vi "ScanCtrl_TE.vi"() -> ()   [LabVIEW 2024]
uses:
  SubVI/GRBL/Status.ctl
  <vilib>/event_ctls.llb/usereventprio.ctl
  <vilib>/ErrorRing/Error Ring.xnode
  SubVI/GRBL/GRBL 1.1.lvlib
panel:
  out "error out":errorcluster
  in  "AutoStartFLIm?":bool
  out "Stage":bool
  in  "Save Button":bool
  in  "RasterScan":bool
  in  "Pre Scan Speed (mm/min)":sgl=3000.0
  in  "Y Pixel Size(mm)":dbl=1.0
  in  "Y distance(mm)":dbl=10.0
  in  "X distance (mm)":dbl=10.0
  in  "Stage COM port":refnum<visa-resource-name>="COM7"
  in  "Tab Control":enum32{"Stage Control", "Stage Setting"}(tab)
  out "Scan Origin MPos":cluster{"X":sgl, "Y":sgl, "Z":sgl}
  in  "Set Origin":bool
  in  "Jog Step Size(mm)":dbl=5.0
  in  "Z--":bool
  in  "Z++":bool
  in  "Y--":bool
  in  "Y++":bool
  in  "X--":bool
  in  "X++":bool
  in  "Hault":bool
  in  "Home":bool
  in  "GoToZero":bool
  out "Current Machine Pos":cluster{"X":sgl, "Y":sgl, "Z":sgl}
  in  "Poll grbl position?":bool
  out "Stage Home MPos":cluster{"X":sgl, "Y":sgl, "Z":sgl}
  in  "X-Axis configuration":T1={"Travel resolution\t(step/mm)"=160.0, "Maximum rate\t(mm/min)"=6000, "Acceleration\t(mm/sec^2)"=1000, "Maximum travel\t(mm)"=160}
  in  "Y-Axis configuration":T1={"Travel resolution\t(step/mm)"=160.0, "Maximum rate\t(mm/min)"=2000, "Acceleration\t(mm/sec^2)"=250, "Maximum travel\t(mm)"=160}
  in  "Z-Axis configuration":T1={"Travel resolution\t(step/mm)"=160.0, "Maximum rate\t(mm/min)"=2000, "Acceleration\t(mm/sec^2)"=250, "Maximum travel\t(mm)"=160}
  out "Current Config":string="$0=10\r\n$1=255\r\n$2=0\r\n$3=0\r\n$4=0\r\n$5=1\r\n$6=0\r\n$10=1\r\n$11=0.010\r\n$12=1000.000\r\n$13=0\r\n$20=1\r\n$21=0\r\n$22=1\r\n$23=0\r\n$24=5.000\r\n$25=3000.000\r\n$26=25\r\n$27=2.000\r\n$30=12000\r\n$31=4000\r\n$32=0\r\n$100=13.333\r\n$101=13.333\r\n$102=98.000\r\n$110=50000.000\r\n$111=50000.000\r\n$112=1800.000\r\n$120=250.000\r\n$121=250.000\r\n$122=50.000\r\n$130=267.000\r\n$131=472.000\r\n$132=68.000\r\nok\r\nok\r\n"
  out "Version information":string="[VER:1.1f.20170324:]\r\n[OPT:VM,15,128]\r\nok\r\nok\r\n"
  in  "Quit":bool
  # "3D Profile Scan Setting"
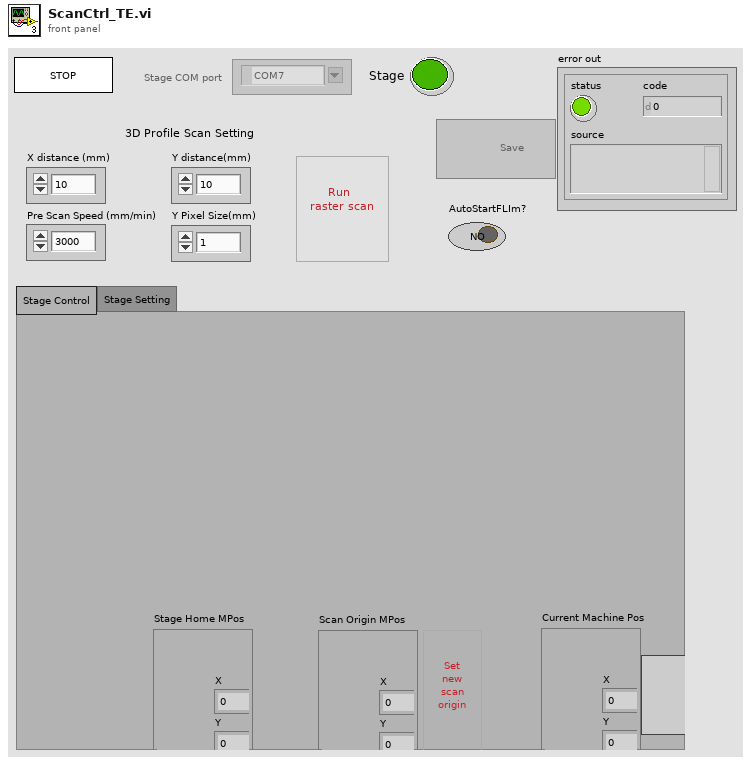
[diagram p1: front panel]
types:
  T1 = cluster{"Travel resolution\t(step/mm)":sgl, "Maximum rate\t(mm/min)":u32, "Acceleration\t(mm/sec^2)":u32, "Maximum travel\t(mm)":u32}
  T2 = typedef "usereventprio.ctl" = enum32{"high priority", "normal priority"}
  T3 = typedef "GRBL 1.1.lvlib/Status.ctl" = enum16{"", "Alarm", "Idle", "Run", "Home"}
  T4 = enum32{"Invalid", "Standard", "Closed", "Hidden", "Minimized", "Maximized"}
  T5 = enum32{"invalid app kind", "Development System", "Run Time System", "Student Edition", "Embedded LabVIEW", "Evaluation", "Custom"}
  T6 = cluster{"Core":cluster{"Current VI Reference":refnum<vi>, "Close Panel on Exit?":bool}, "StageStatus":bool, "StageCOM":refnum<visa-resource-name>, "StepSize":dbl, "ScanOrigin":cluster{"X":sgl, "Y":sgl, "Z":sgl}, "HomeMposOrigin":cluster{"X":sgl, "Y":sgl, "Z":sgl}, "Tic":i32, "YPixelSize(mm)":dbl, "StageHomed?":bool, "SaveFilePath":path}
  T7 = cluster{"remote start event":refnum<user-event>, "remote stop event":refnum<user-event>}
  T8 = cluster{"Current VI Reference":refnum<vi>, "Close Panel on Exit?":bool}
  T9 = enum8{"Enabled", "Disabled", "Disabled and Grayed Out"}
  T10 = cluster{"Invert enable pin":bool, "Invert limit pin":bool, "Invert probe pin":bool}
  T11 = cluster{"Reverse X":bool, "Reverse Y":bool, "Reverse Z":bool}
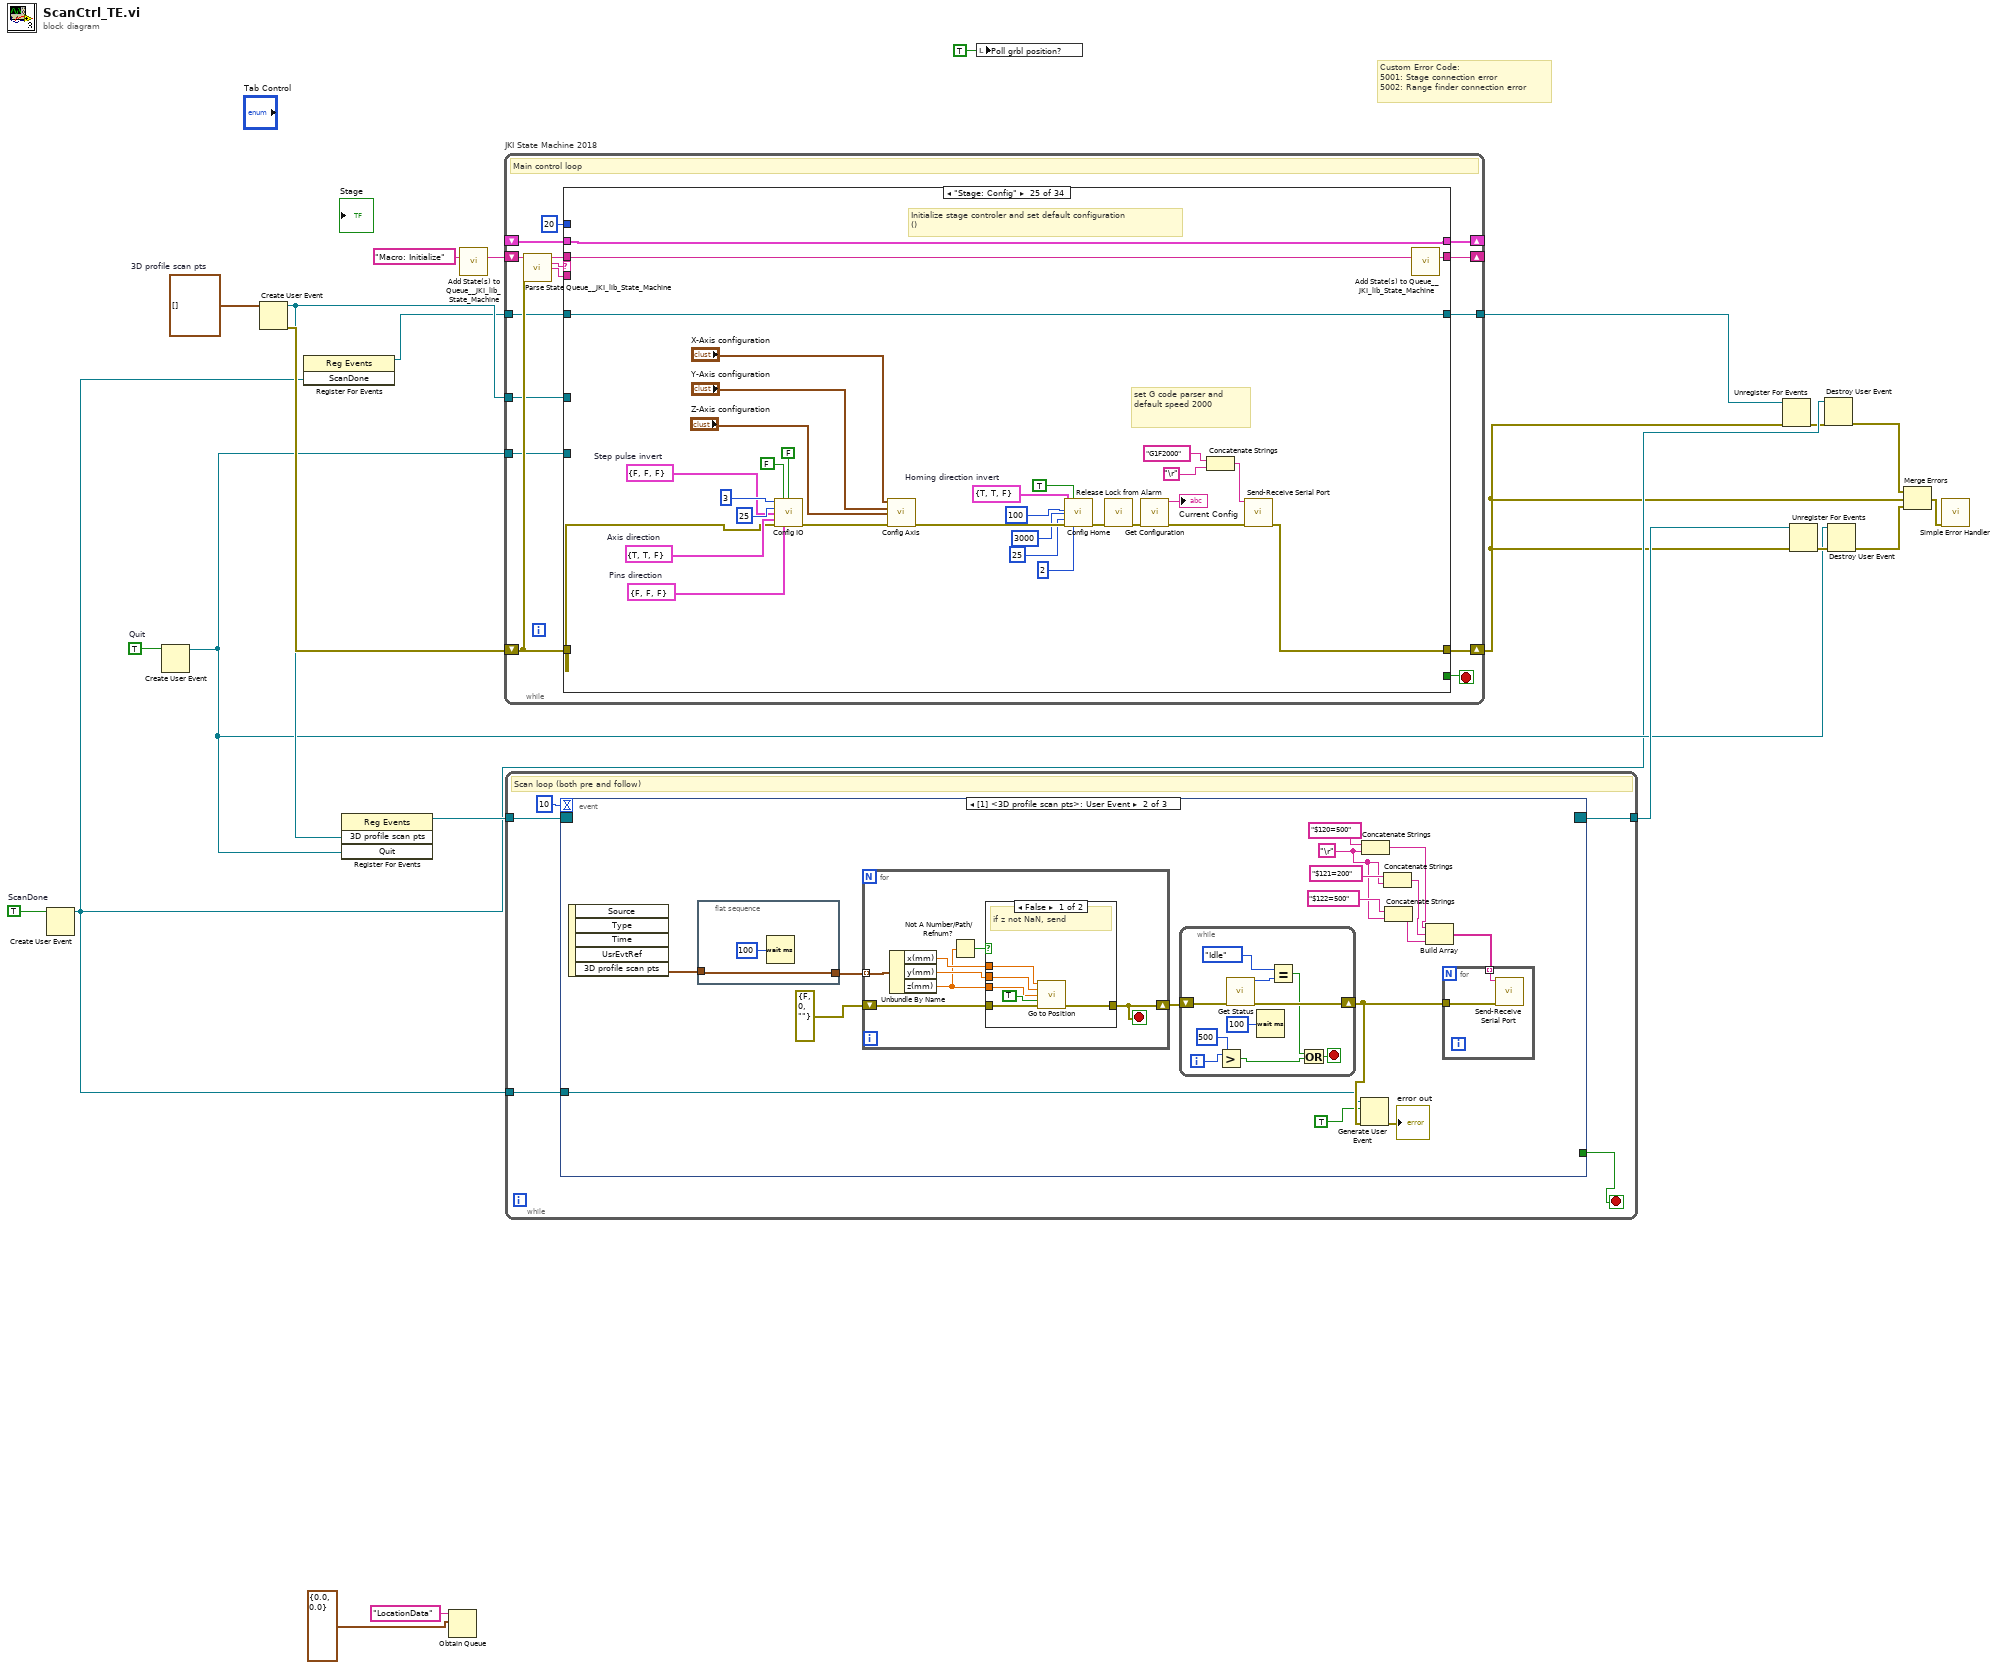
[diagram p0: block diagram]
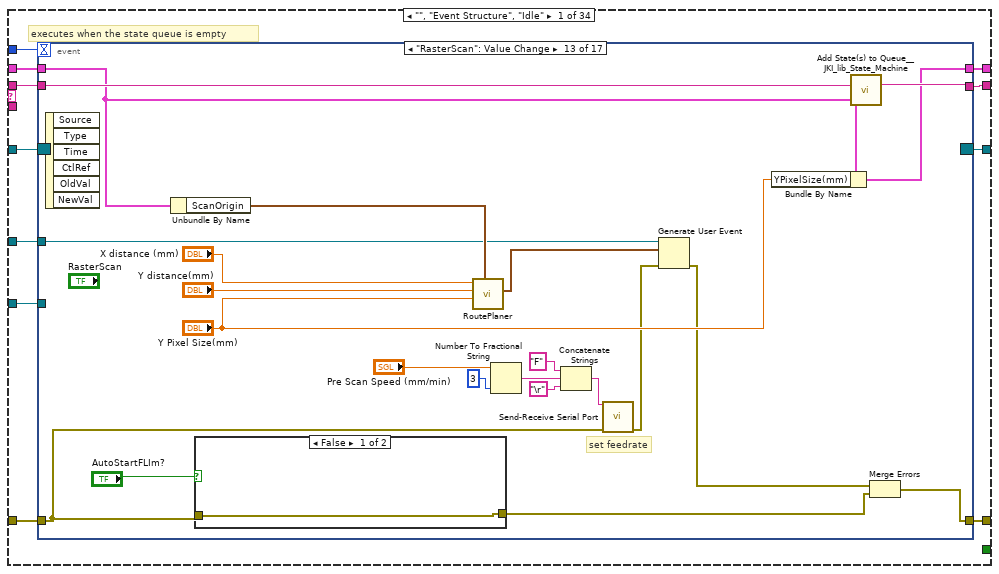
[diagram p2: hidden frame]
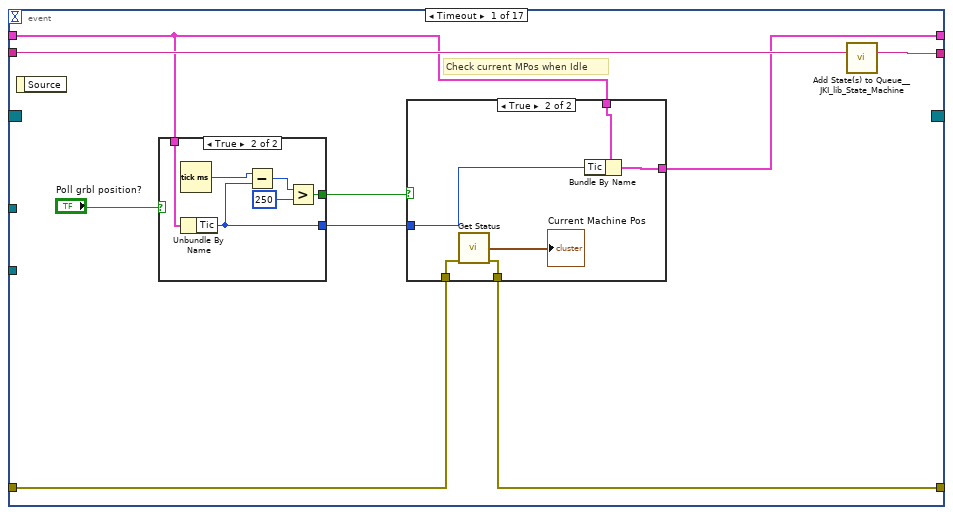
[diagram p3: hidden frame]
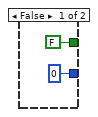
[diagram p4: hidden frame]
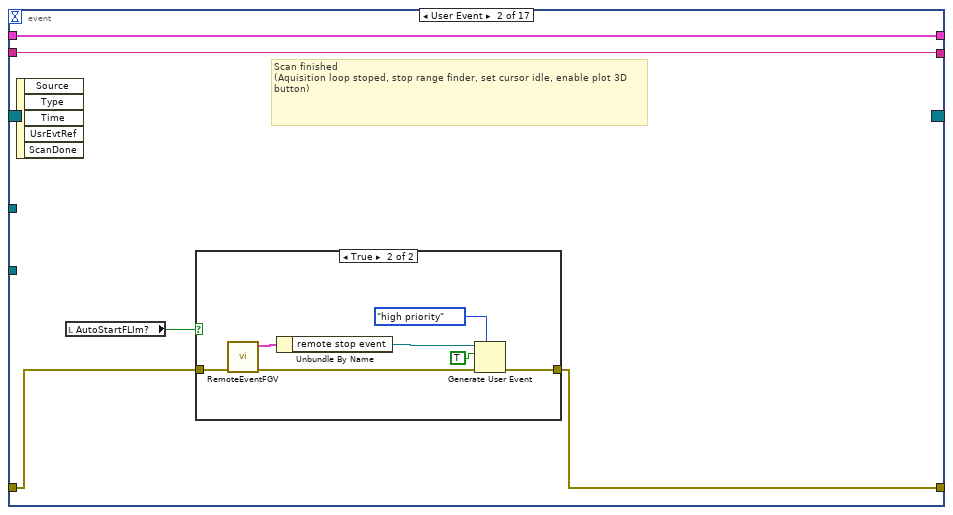
[diagram p6: hidden frame]
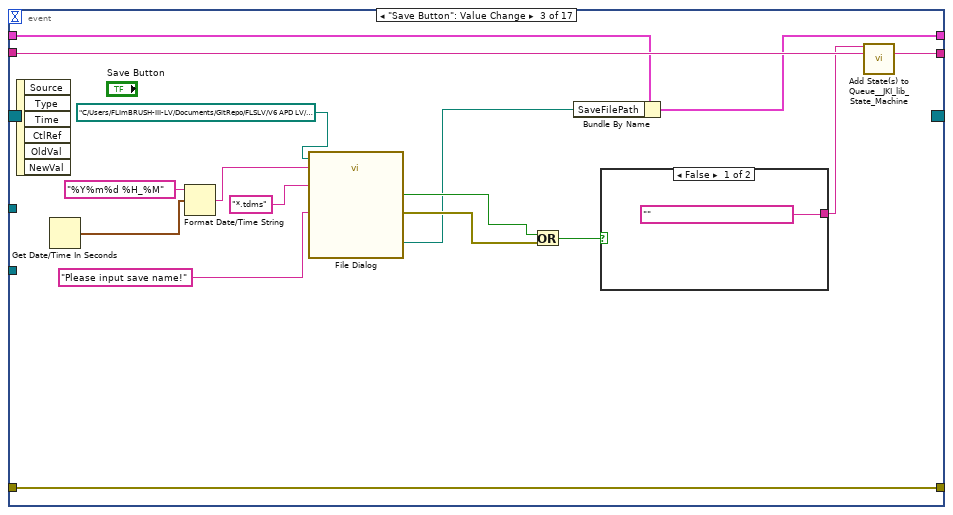
[diagram p8: hidden frame]
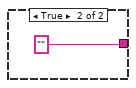
[diagram p9: hidden frame]
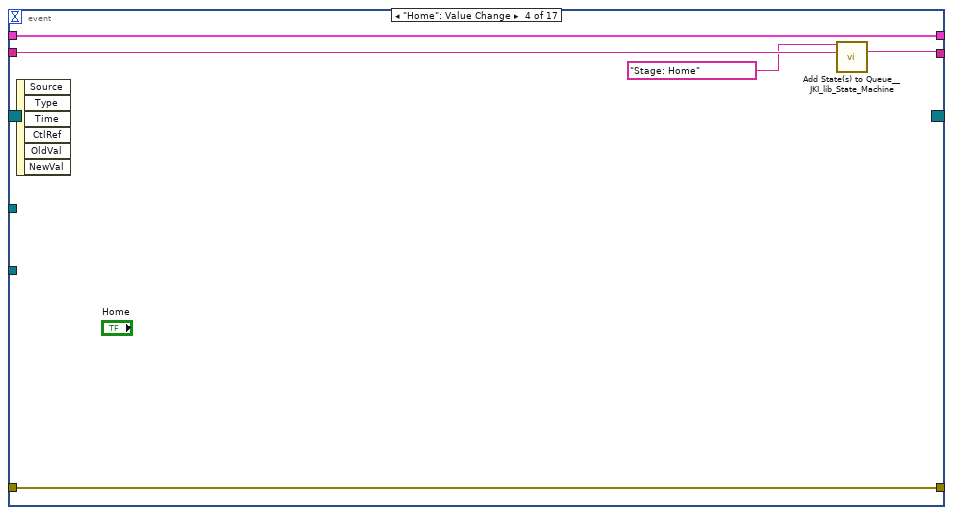
[diagram p10: hidden frame]
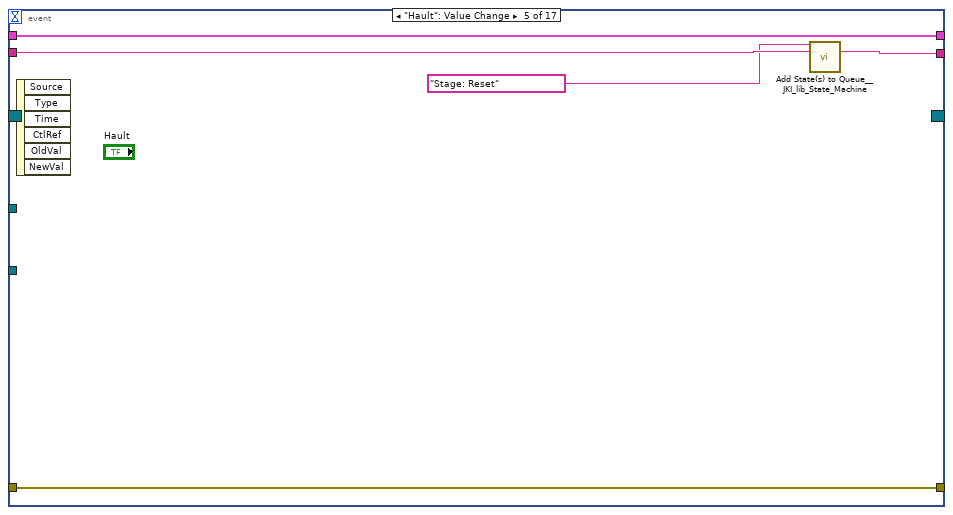
[diagram p11: hidden frame]
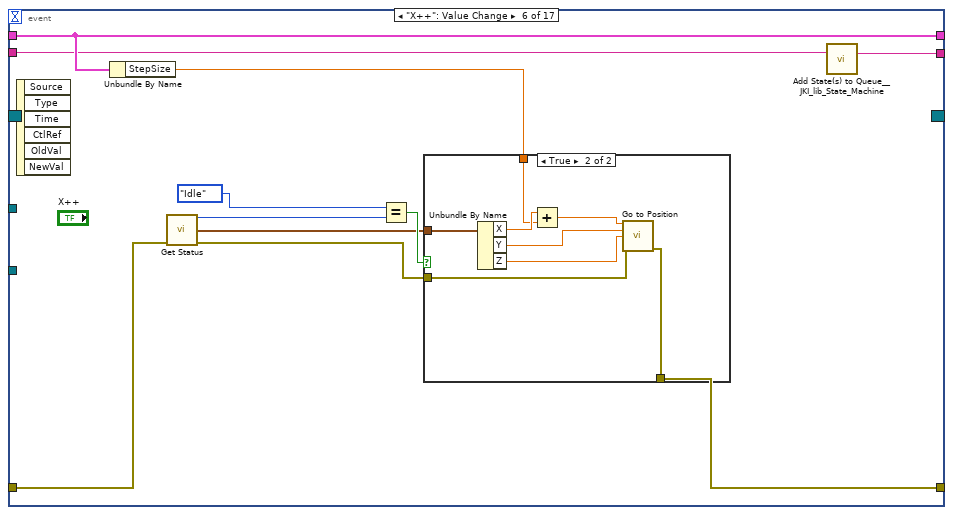
[diagram p12: hidden frame]
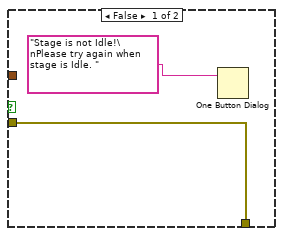
[diagram p13: hidden frame]
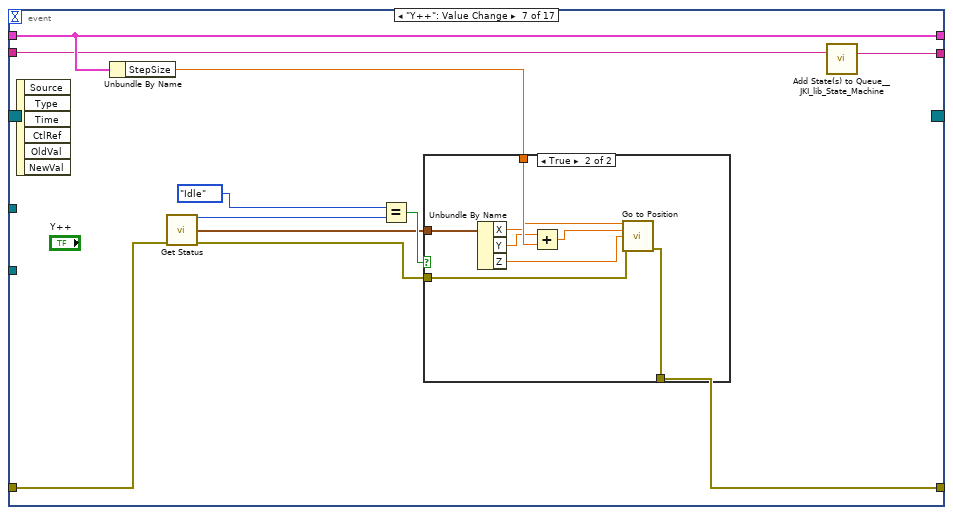
[diagram p14: hidden frame]
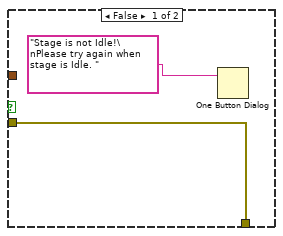
[diagram p15: hidden frame]
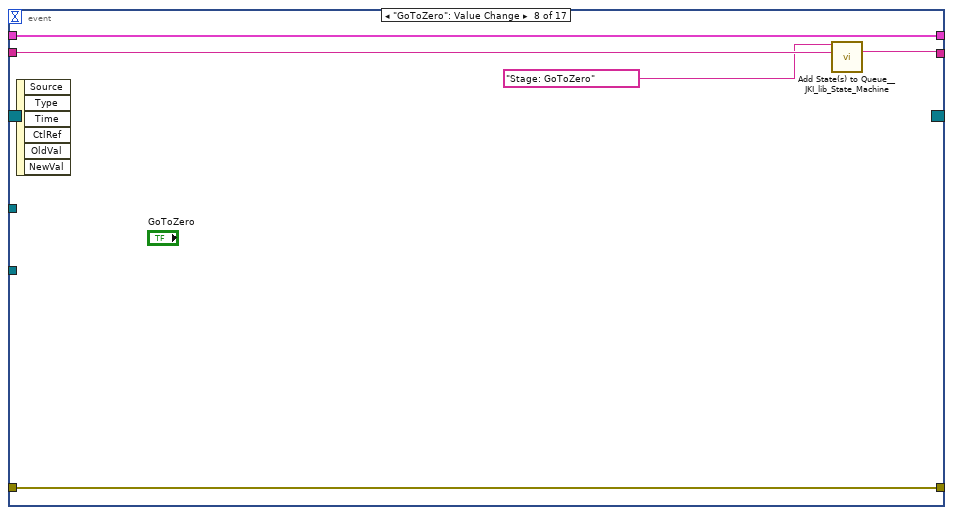
[diagram p16: hidden frame]
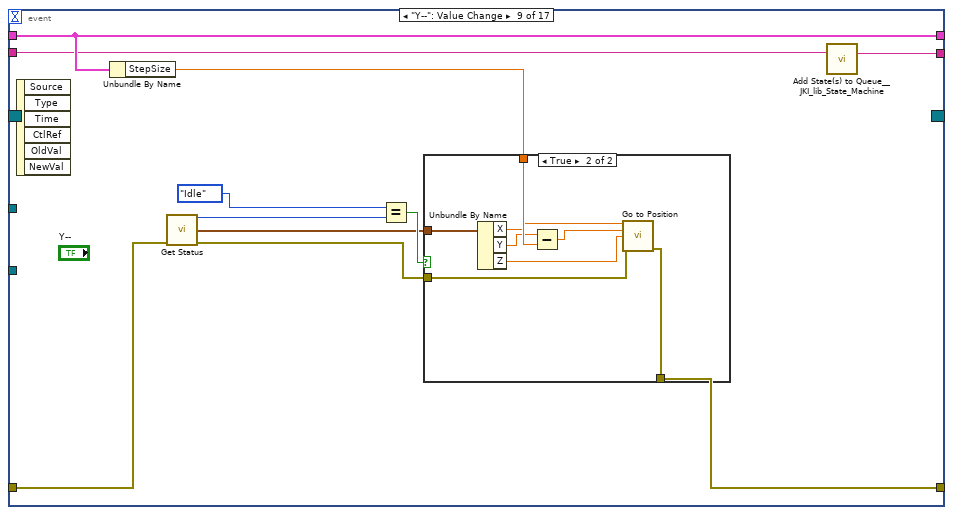
[diagram p17: hidden frame]
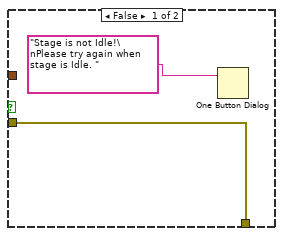
[diagram p18: hidden frame]
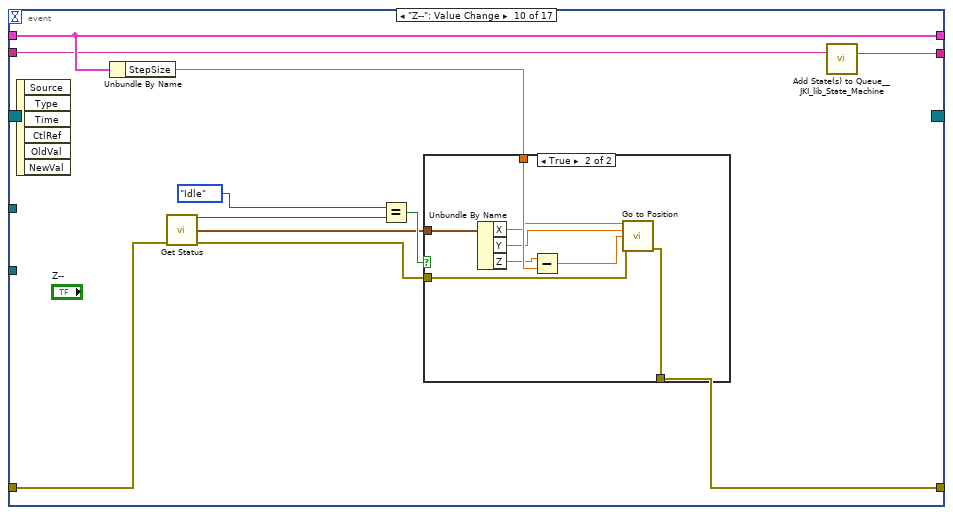
[diagram p19: hidden frame]
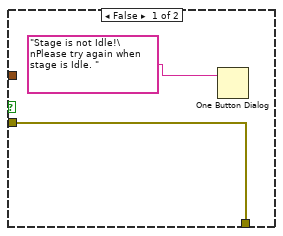
[diagram p20: hidden frame]
diagram:
  w9 = TRUE  # ScanDone
  w15 = TRUE  # Quit
  w16 = cluster{"x(mm)":dbl, "y(mm)":dbl, "z(mm)":dbl}[] []  # 3D profile scan pts
  # "Custom Error Code:\n5001: Stage connection error\n5002: Range finder connection error"
  n1 = Create User Event(user event datatype=w9) -> (user event=w6:refnum<user-event>)  [unwired: 1 in, 1 out]
  n2 = Create User Event(user event datatype=w15) -> (user event=w10:refnum<user-event>)  [unwired: 1 in, 1 out]
  n3 = Create User Event(user event datatype=w16) -> (user event=w18:refnum<user-event>, error out=w19:errorcluster)  [unwired: 1 in]
  n4 = register-events(w6) -> (reference out=w8:refnum<event-registration>)  [unwired: 2 in, 1 out]
  n5 = register-events(w18, w10) -> (reference out=w14:refnum<event-registration>)  [unwired: 2 in, 1 out]
  n6 = Obtain Queue(name (unnamed)="LocationData", element data type=cluster{"Time":dbl, "x":dbl} {"Time"=0.0, "x"=0.0}) -> ()  [unwired: 3 in, 3 out]
  n7 = call <vilib>:"Add State(s) to Queue__JKI_lib_State_Machine.vi"("State(s) in (\"\")"="Macro: Initialize") -> ("States Out"=w22:string)  [unwired: 14 in]
  n8 = while "JKI State Machine 2018" {
    shift-right: [w32] -> _
    shift-left: _ -> [w23]
    shift-right: [w35] -> w1
    shift-left: w19 -> [w30]
    shift-right: [w34] -> _
    shift-left: w22 -> [w29]
    tunnel: w18 -> [w28]
    tunnel: w10 -> [w27]
    tunnel: w8 -> [w25]
    tunnel: [w24] -> w7
    stop <- w33 stop-if-true
    # "Main control loop"
    n9 = call <vilib>:"Parse State Queue__JKI_lib_State_Machine.vi"("State Queue"=w29, "Error In (no error)"=w30) -> ("Remaining States"=w37:string, "Current State"=w26:string, "Arguments"=w36:string)  [unwired: 11 in]
    n10 = case shown="\"Stage: Config\"" w26 {
      selector: w26 -> [_ _ _ _ _ w326 _ _ _ _ _ _ _ _ _ _ _ _ _ _ _ _ _ _ _ _ _ _ _ _ _ _ _ _]
      tunnel: w37 -> [w48 w301 w302 w319 w324 w330 w350 w357 w366 w371 w386 w393 w400 w405 w412 w418 w423 w430 w437 w444 w456 w526 w538 w556 w587 w598 w621 w662 w670 w682 w689 w694 w699 w704]
      tunnel: w36 -> [_ _ _ _ _ _ _ _ _ _ _ _ _ _ _ _ _ _ _ w439 w450 _ _ _ _ _ _ w657 _ _ w685 _ _ _]
      tunnel: w23 -> [w46 w298 w305 w316 w321 w328 w343 w354 w364 w368 _ w389 w395 w402 w409 w415 w420 w427 w435 w442 w452 w523 w528 w554 w568 w594 w615 w660 w664 w679 w686 w691 w696 w701]
      tunnel: [w45 w299 w306 w317 w322 w332 w347 errorcluster {"status"=FALSE, "code"=0, "source"=""} ("error out") w360 w369 w383 w391 w396 w403 w410 w416 w421 w428 w434 w440 w453 w524 w532 w553 w562 w596 w618 w659 w668 w680 w687 w692 w697 w702] -> w35
      tunnel: w30 -> [w44 w299 w306 w317 w322 w331 w347 w353 w359 w369 w383 w391 w397 w403 w410 w416 w421 w428 w434 w441 w454 w524 w536 w552 w567 w592 w619 w658 w667 w680 w687 w692 w697 w702]
      tunnel: [w47 w300 w307 w318 w323 w329 w349 w356 w365 w370 w385 w392 w399 w404 w411 w417 w422 w429 w436 w443 w455 w525 w537 w555 w586 w597 w620 w661 w669 w681 w688 w693 w698 w703] -> w34
      tunnel: [_ _ _ _ _ _ _ _ TRUE _ _ _ _ _ _ _ _ _ _ _ _ _ _ _ _ _ _ _ _ _ _ _ _ _] -> w33
      tunnel: [w43 w298 w305 w316 w321 w328 w348 w354 w364 w368 w384 w390 w395 w402 w409 w415 w420 w427 w435 w442 w452 w523 w535 w554 w568 w595 w617 w660 w666 w679 w686 w691 w696 w701] -> w32
      tunnel: 20 ("Timeout") -> [w42 _ _ _ _ _ _ _ _ _ _ _ _ _ _ _ _ _ _ _ _ _ _ _ _ _ _ _ _ _ _ _ _ _]
      tunnel: w28 -> [w41 _ _ _ _ _ _ _ _ _ _ _ _ _ _ _ _ _ _ _ _ _ _ _ _ _ _ _ _ _ _ _ _ _]
      tunnel: w27 -> [w40 _ _ _ _ _ _ _ w361 _ _ _ _ _ _ _ _ _ _ _ _ _ _ _ _ _ _ _ _ _ _ _ _ _]
      tunnel: w25 -> [w39 w297 w303 w308 w320 w325 w337 w351 w358 w367 w374 w387 w394 w401 w408 w414 w419 w426 w433 w438 w449 w522 w530 w551 w558 w593 w616 w656 w665 w678 w683 w690 w695 w700]
      tunnel: [w38 w297 w303 w308 w320 w325 w337 w351 w358 w367 w374 w387 w394 w401 w408 w414 w419 w426 w433 w438 w449 w522 w530 w551 w558 w593 w616 w656 w665 w678 w683 w690 w695 w700] -> w24
      frame "", "Event Structure", "Idle" {
        # "executes when the state queue is empty"
        n11 = event shown="[12] \"RasterScan\": Value Change" {
          selector: w39 -> [_ _ _ _ _ _ _ _ _ _ _ _ _ _ _ _ _]
          dyn-events: [_ _ _ _ _ _ _ _ _ _ _ _ _ _ _ _ _] -> w38
          timeout: w42 -> [_ _ _ _ _ _ _ _ _ _ _ _ _ _ _ _ _]
          tunnel: w48 -> [w57 w77 w100 w107 w113 w123 w144 w158 w170 w191 w212 w227 w249 w268 w283 w290 w296]
          tunnel: [w56 w77 w101 w108 w112 w124 w145 w159 w171 w192 w213 w227 w248 w269 w283 w289 w295] -> w47
          tunnel: w46 -> [w51 w78 w93 w109 w114 w125 w146 w161 w172 w193 w214 w230 w240 w270 w285 w288 w293]
          tunnel: [w55 w75 w102 w106 w110 w116 w137 w160 w163 w184 w205 w225 w233 w261 w281 w286 w294] -> w45
          tunnel: w44 -> [w54 w76 w102 w106 w110 w115 w136 w160 w162 w183 w204 w226 w234 w260 w281 w286 w294]
          tunnel: [w52 w78 w92 w109 w114 w125 w146 w161 w172 w193 w214 w229 w241 w270 w284 w288 w293] -> w43
          tunnel: w41 -> [_ _ _ _ _ _ _ _ _ _ _ _ w238 _ _ _ _]
          tunnel: w40 -> [_ _ _ _ _ _ _ _ _ _ _ _ _ _ _ _ _]
          event Timeout {
            # "Check current MPos when Idle"
            n12 = event-data() -> ()  [unwired: 1 in, 1 out]
            n13 = case shown="True" "Poll grbl position?" {
              tunnel: [FALSE w62] -> w53
              tunnel: w51 -> [_ w61]
              tunnel: [0 ("Tic") w60] -> w50
              frame False {
              }
              frame True {
                n14 = Tick Count (ms)() -> (millisecond timer value=w65:u32)
                n15 = Unbundle By Name(w61) -> ("Tic"=w60:i32)
                n16 = Subtract(x=w65, y=w60) -> (x-y=w64:u32)
                n17 = Greater?(x=w64, y=u32 250) -> (0:w62:bool)
              }
            }
            n18 = case shown="True" w53 {
              tunnel: [w67 w73] -> w55
              tunnel: w54 -> [w67 w72]
              tunnel: w51 -> [w66 w70]
              tunnel: [w66 w69] -> w52
              tunnel: w50 -> [_ w68]
              frame False {
              }
              frame True {
                n19 = call "Get Status.vi"("error in (no error)"=w72) -> ("Current position"=→"Current Machine Pos":cluster{"X":sgl, "Y":sgl, "Z":sgl}, "error out"=w73:errorcluster)  [unwired: 10 in, 3 out]
                n20 = Bundle By Name(cluster=w70, "Tic"=w68) -> (w69:T6)
              }
            }
            n21 = call <vilib>:"Add State(s) to Queue__JKI_lib_State_Machine.vi"("State(s) in (\"\")"=w57) -> ("States Out"=w56:string)  [unwired: 14 in]
          }
          event User Event {
            # "Scan finished\n(Aquisition loop stoped, stop range finder, set cursor idle, enable plot 3D button)"
            n22 = event-data() -> ()  [unwired: 1 in, 5 out]
            n23 = local read "AutoStartFLIm?"() -> (w74:bool)
            n24 = case shown="True" w74 {
              tunnel: w76 -> [w79 w81]
              tunnel: [w79 w80] -> w75
              frame False {
              }
              frame True {
                n25 = call "RemoteEventFGV.vi"("Error In"=w81) -> ("Error Out"=w83:errorcluster, "Remote Event out"=w86:T7)  [unwired: 9 in]
                n26 = Unbundle By Name(w86) -> ("remote stop event"=w85:refnum<user-event>)
                n27 = Generate User Event(priority (normal)=usereventprio."high priority", user event=w85, event data cluster=TRUE ("event data"), error in=w83) -> (error out=w80:errorcluster)  [unwired: 1 out]
              }
            }
          }
          event "Save Button": Value Change {
            n28 = event-data() -> ()  [unwired: 1 in, 6 out]
            n29 = Get Date/Time In Seconds() -> (seconds since 1Jan1904=w89:timestamp)
            n30 = Format Date/Time String(time format string (%c)="%Y%m%d %H_%M", seconds (now)=w89) -> (date/time string=w87:string)  [unwired: 1 in]
            n31 = call "File Dialog"("start path"=path "C:/Users/FLImBRUSH-III-LV/Documents/GitRepo/FLSLV/V6 APD LV/Data", "prompt"="Please input save name!", "default name"=w87, "pattern (all files)"="*.tdms") -> ("selected path"=w91:path, "cancelled"=w96:bool, "error out"=w95:errorcluster)  [unwired: 8 in, 1 out]
            n32 = Or(x=w96, y=w95) -> (x .or. y?=w94:bool)
            n33 = Bundle By Name(cluster=w93, "SaveFilePath"=w91) -> (w92:T6)
            n34 = case shown="False" w94 {
              tunnel: ["" ("State(s) in Front (\"\")") "" ("State(s) in Front (\"\")")] -> w97
              frame False {
              }
              frame True {
              }
            }
            n35 = call <vilib>:"Add State(s) to Queue__JKI_lib_State_Machine.vi"("State(s) in Front (\"\")"=w97, "State(s) in (\"\")"=w100) -> ("States Out"=w101:string)  [unwired: 13 in]
          }
          event "Home": Value Change {
            n36 = event-data() -> ()  [unwired: 1 in, 6 out]
            n37 = call <vilib>:"Add State(s) to Queue__JKI_lib_State_Machine.vi"("State(s) in Front (\"\")"="Stage: Home" ("State(s) in Front (\"\")"), "State(s) in (\"\")"=w107) -> ("States Out"=w108:string)  [unwired: 13 in]
          }
          event "Hault": Value Change {
            n38 = event-data() -> ()  [unwired: 1 in, 6 out]
            n39 = call <vilib>:"Add State(s) to Queue__JKI_lib_State_Machine.vi"("State(s) in Front (\"\")"="Stage: Reset" ("State(s) in Front (\"\")"), "State(s) in (\"\")"=w113) -> ("States Out"=w112:string)  [unwired: 13 in]
          }
          event "X++": Value Change {
            n40 = event-data() -> ()  [unwired: 1 in, 6 out]
            n41 = Unbundle By Name(w125) -> ("StepSize"=w118:dbl)
            n42 = call "Get Status.vi"("error in (no error)"=w115) -> ("Status"=w122:T3, "Current position"=w119:cluster{"X":sgl, "Y":sgl, "Z":sgl}, "error out"=w117:errorcluster)  [unwired: 10 in, 2 out]
            n43 = Equal?(x=Status."Idle" ("Status"), y=w122) -> (x = y?=w120:bool)
            n44 = case shown="True" w120 {
              tunnel: w119 -> [_ w135]
              tunnel: w118 -> [_ w128]
              tunnel: w117 -> [w127 w131]
              tunnel: [w127 w130] -> w116
              frame False {
                n45 = One Button Dialog(message="Stage is not Idle!\nPlease try again when stage is Idle. ") -> ()  [unwired: 1 in, 1 out]
              }
              frame True {
                n46 = Unbundle By Name(w135) -> ("X"=w129:sgl, "Y"=w133:sgl, "Z"=w132:sgl)
                n47 = Add(x=w129, y=w128) -> (x+y=w134:dbl)
                n48 = call "Go to Position.vi"("X (mm)"=w134, "Y (mm)"=w133, "Z (mm)"=w132, "error in (no error)"=w131) -> ("error out"=w130:errorcluster)  [unwired: 11 in]
              }
            }
            n49 = call <vilib>:"Add State(s) to Queue__JKI_lib_State_Machine.vi"("State(s) in (\"\")"=w123) -> ("States Out"=w124:string)  [unwired: 14 in]
          }
          event "Y++": Value Change {
            n50 = event-data() -> ()  [unwired: 1 in, 6 out]
            n51 = Unbundle By Name(w146) -> ("StepSize"=w139:dbl)
            n52 = call "Get Status.vi"("error in (no error)"=w136) -> ("Status"=w143:T3, "Current position"=w140:cluster{"X":sgl, "Y":sgl, "Z":sgl}, "error out"=w138:errorcluster)  [unwired: 10 in, 2 out]
            n53 = Equal?(x=Status."Idle" ("Status"), y=w143) -> (x = y?=w141:bool)
            n54 = case shown="True" w141 {
              tunnel: w140 -> [_ w156]
              tunnel: w139 -> [_ w152]
              tunnel: w138 -> [w148 w154]
              tunnel: [w148 w153] -> w137
              frame False {
                n55 = One Button Dialog(message="Stage is not Idle!\nPlease try again when stage is Idle. ") -> ()  [unwired: 1 in, 1 out]
              }
              frame True {
                n56 = Unbundle By Name(w156) -> ("X"=w149:sgl, "Y"=w151:sgl, "Z"=w155:sgl)
                n57 = Add(x=w151, y=w152) -> (x+y=w150:dbl)
                n58 = call "Go to Position.vi"("X (mm)"=w149, "Y (mm)"=w150, "Z (mm)"=w155, "error in (no error)"=w154) -> ("error out"=w153:errorcluster)  [unwired: 11 in]
              }
            }
            n59 = call <vilib>:"Add State(s) to Queue__JKI_lib_State_Machine.vi"("State(s) in (\"\")"=w144) -> ("States Out"=w145:string)  [unwired: 14 in]
          }
          event "GoToZero": Value Change {
            n60 = event-data() -> ()  [unwired: 1 in, 6 out]
            n61 = call <vilib>:"Add State(s) to Queue__JKI_lib_State_Machine.vi"("State(s) in Front (\"\")"="Stage: GoToZero" ("State(s) in Front (\"\")"), "State(s) in (\"\")"=w158) -> ("States Out"=w159:string)  [unwired: 13 in]
          }
          event "Y--": Value Change {
            n62 = event-data() -> ()  [unwired: 1 in, 6 out]
            n63 = Unbundle By Name(w172) -> ("StepSize"=w165:dbl)
            n64 = call "Get Status.vi"("error in (no error)"=w162) -> ("Status"=w169:T3, "Current position"=w166:cluster{"X":sgl, "Y":sgl, "Z":sgl}, "error out"=w164:errorcluster)  [unwired: 10 in, 2 out]
            n65 = Equal?(x=Status."Idle" ("Status"), y=w169) -> (x = y?=w167:bool)
            n66 = case shown="True" w167 {
              tunnel: w166 -> [_ w182]
              tunnel: w165 -> [_ w178]
              tunnel: w164 -> [w174 w180]
              tunnel: [w174 w179] -> w163
              frame False {
                n67 = One Button Dialog(message="Stage is not Idle!\nPlease try again when stage is Idle. ") -> ()  [unwired: 1 in, 1 out]
              }
              frame True {
                n68 = Unbundle By Name(w182) -> ("X"=w175:sgl, "Y"=w177:sgl, "Z"=w181:sgl)
                n69 = Subtract(x=w177, y=w178) -> (x-y=w176:dbl)
                n70 = call "Go to Position.vi"("X (mm)"=w175, "Y (mm)"=w176, "Z (mm)"=w181, "error in (no error)"=w180) -> ("error out"=w179:errorcluster)  [unwired: 11 in]
              }
            }
            n71 = call <vilib>:"Add State(s) to Queue__JKI_lib_State_Machine.vi"("State(s) in (\"\")"=w170) -> ("States Out"=w171:string)  [unwired: 14 in]
          }
          event "Z--": Value Change {
            n72 = event-data() -> ()  [unwired: 1 in, 6 out]
            n73 = Unbundle By Name(w193) -> ("StepSize"=w186:dbl)
            n74 = call "Get Status.vi"("error in (no error)"=w183) -> ("Status"=w190:T3, "Current position"=w187:cluster{"X":sgl, "Y":sgl, "Z":sgl}, "error out"=w185:errorcluster)  [unwired: 10 in, 2 out]
            n75 = Equal?(x=Status."Idle" ("Status"), y=w190) -> (x = y?=w188:bool)
            n76 = case shown="True" w188 {
              tunnel: w187 -> [_ w203]
              tunnel: w186 -> [_ w200]
              tunnel: w185 -> [w195 w202]
              tunnel: [w195 w201] -> w184
              frame False {
                n77 = One Button Dialog(message="Stage is not Idle!\nPlease try again when stage is Idle. ") -> ()  [unwired: 1 in, 1 out]
              }
              frame True {
                n78 = Unbundle By Name(w203) -> ("X"=w199:sgl, "Y"=w198:sgl, "Z"=w196:sgl)
                n79 = Subtract(x=w196, y=w200) -> (x-y=w197:dbl)
                n80 = call "Go to Position.vi"("X (mm)"=w199, "Y (mm)"=w198, "Z (mm)"=w197, "error in (no error)"=w202) -> ("error out"=w201:errorcluster)  [unwired: 11 in]
              }
            }
            n81 = call <vilib>:"Add State(s) to Queue__JKI_lib_State_Machine.vi"("State(s) in (\"\")"=w191) -> ("States Out"=w192:string)  [unwired: 14 in]
          }
          event "Z++": Value Change {
            n82 = event-data() -> ()  [unwired: 1 in, 6 out]
            n83 = Unbundle By Name(w214) -> ("StepSize"=w207:dbl)
            n84 = call "Get Status.vi"("error in (no error)"=w204) -> ("Status"=w211:T3, "Current position"=w208:cluster{"X":sgl, "Y":sgl, "Z":sgl}, "error out"=w206:errorcluster)  [unwired: 10 in, 2 out]
            n85 = Equal?(x=Status."Idle" ("Status"), y=w211) -> (x = y?=w209:bool)
            n86 = case shown="True" w209 {
              tunnel: w208 -> [_ w224]
              tunnel: w207 -> [_ w221]
              tunnel: w206 -> [w216 w223]
              tunnel: [w216 w222] -> w205
              frame False {
                n87 = One Button Dialog(message="Stage is not Idle!\nPlease try again when stage is Idle. ") -> ()  [unwired: 1 in, 1 out]
              }
              frame True {
                n88 = Unbundle By Name(w224) -> ("X"=w220:sgl, "Y"=w219:sgl, "Z"=w217:sgl)
                n89 = Add(x=w217, y=w221) -> (x+y=w218:dbl)
                n90 = call "Go to Position.vi"("X (mm)"=w220, "Y (mm)"=w219, "Z (mm)"=w218, "error in (no error)"=w223) -> ("error out"=w222:errorcluster)  [unwired: 11 in]
              }
            }
            n91 = call <vilib>:"Add State(s) to Queue__JKI_lib_State_Machine.vi"("State(s) in (\"\")"=w212) -> ("States Out"=w213:string)  [unwired: 14 in]
          }
          event "Set Origin": Value Change {
            # "reset encoder"
            n92 = event-data() -> ()  [unwired: 1 in, 6 out]
            n93 = call "Get Status.vi"("error in (no error)"=w226) -> ("Current position"=w228:cluster{"X":sgl, "Y":sgl, "Z":sgl}, "error out"=w225:errorcluster)  [unwired: 10 in, 3 out]
            "Scan Origin MPos" <- w228
            n94 = Bundle By Name(cluster=w230, "ScanOrigin"=w228) -> (w229:T6)
          }
          event "RasterScan": Value Change {
            # "set feedrate"
            n95 = event-data() -> ()  [unwired: 1 in, 6 out]
            n96 = Unbundle By Name(w240) -> ("ScanOrigin"=w250:cluster{"X":sgl, "Y":sgl, "Z":sgl})
            n97 = case shown="False" "AutoStartFLIm?" {
              tunnel: w234 -> [w253 w255]
              tunnel: [w253 w254] -> w232
              frame False {
              }
              frame True {
                n98 = call "RemoteEventFGV.vi"() -> ("Remote Event out"=w259:T7)  [unwired: 10 in, 1 out]
                n99 = Unbundle By Name(w259) -> ("remote start event"=w258:refnum<user-event>)
                n100 = Generate User Event(priority (normal)=usereventprio."high priority", user event=w258, event data cluster=TRUE ("event data"), error in=w255) -> (error out=w254:errorcluster)  [unwired: 1 out]
              }
            }
            n101 = call "RoutePlaner.vi"("Origin In"=w250, "Pixel Size(mm)"="Y Pixel Size(mm)", "Y distance(mm)"="Y distance(mm)", "X distance (mm)"="X distance (mm)") -> ("PtArray"=w237:cluster{"x":dbl, "y":dbl, "z":dbl}[])  [unwired: 5 in, 2 out]
            n102 = Number To Fractional String(number="Pre Scan Speed (mm/min)", precision (6)=i16 3) -> (F-format string=w244:string)  [unwired: 2 in]
            n103 = Concatenate Strings("F" ("string"), w244, "\r") -> (w243:string)
            n104 = call "Send-Receive Serial Port.vi"("Data to write"=w243, "error in (no error)"=w234) -> ("error out"=w236:errorcluster)  [unwired: 12 in, 1 out]
            n105 = Generate User Event(user event=w238, event data cluster=w237, error in=w236) -> (error out=w235:errorcluster)  [unwired: 1 in, 1 out]
            n106 = Bundle By Name(cluster=w240, "YPixelSize(mm)"="Y Pixel Size(mm)") -> (w241:T6)
            n107 = call <vilib>:"Add State(s) to Queue__JKI_lib_State_Machine.vi"("State(s) in (\"\")"=w249) -> ("States Out"=w248:string)  [unwired: 14 in]
            n108 = Merge Errors(w235, w232) -> (w233:errorcluster)
          }
          event "X--": Value Change {
            n109 = event-data() -> ()  [unwired: 1 in, 6 out]
            n110 = Unbundle By Name(w270) -> ("StepSize"=w263:dbl)
            n111 = call "Get Status.vi"("error in (no error)"=w260) -> ("Status"=w267:T3, "Current position"=w264:cluster{"X":sgl, "Y":sgl, "Z":sgl}, "error out"=w262:errorcluster)  [unwired: 10 in, 2 out]
            n112 = Equal?(x=Status."Idle" ("Status"), y=w267) -> (x = y?=w265:bool)
            n113 = case shown="True" w265 {
              tunnel: w264 -> [_ w280]
              tunnel: w263 -> [_ w274]
              tunnel: w262 -> [w272 w276]
              tunnel: [w272 w275] -> w261
              frame False {
                n114 = One Button Dialog(message="Stage is not Idle!\nPlease try again when stage is Idle. ") -> ()  [unwired: 1 in, 1 out]
              }
              frame True {
                n115 = Unbundle By Name(w280) -> ("X"=w273:sgl, "Y"=w278:sgl, "Z"=w277:sgl)
                n116 = Subtract(x=w273, y=w274) -> (x-y=w279:dbl)
                n117 = call "Go to Position.vi"("X (mm)"=w279, "Y (mm)"=w278, "Z (mm)"=w277, "error in (no error)"=w276) -> ("error out"=w275:errorcluster)  [unwired: 11 in]
              }
            }
            n118 = call <vilib>:"Add State(s) to Queue__JKI_lib_State_Machine.vi"("State(s) in (\"\")"=w268) -> ("States Out"=w269:string)  [unwired: 14 in]
          }
          event "Jog Step Size(mm)": Value Change {
            n119 = event-data() -> ("NewVal"=w282:dbl)  [unwired: 1 in, 5 out]
            n120 = Bundle By Name(cluster=w285, "StepSize"=w282) -> (w284:T6)
          }
          event "Quit": Value Change {
            # "Exit Button Value Change (pressed) Event\n(this executes Macro: Exit to terminate the VI)"
            n121 = event-data() -> ()  [unwired: 1 in, 1 out]
            n122 = call <vilib>:"Add State(s) to Queue__JKI_lib_State_Machine.vi"("State(s) in Front (\"\")"="Macro: Exit", "State(s) in (\"\")"=w290) -> ("States Out"=w289:string)  [unwired: 13 in]
          }
          event Panel Close? {
            # "Discard the event because we'll close the front panel ourselves in Macro: Exit"
            # "Close Panel button (pressed) Event\n(this executes Macro: Exit to terminate the VI)"
            n123 = event-data() -> ()  [unwired: 1 in, 1 out]
            n124 = call <vilib>:"Add State(s) to Queue__JKI_lib_State_Machine.vi"("State(s) in Front (\"\")"="Macro: Exit", "State(s) in (\"\")"=w296) -> ("States Out"=w295:string)  [unwired: 13 in]
            n125 = event-data("Discard?"=TRUE) -> ()  [unwired: 1 in, 1 out]
          }
        }
      }
      frame "---------- Macro ----------" {
        # "Do not put any code in this frame.\n(It is a separator no-op. You can make a copy of this frame to create a new Macro frame)"
        n126 = call <vilib>:"Add State(s) to Queue__JKI_lib_State_Machine.vi"("State(s) in (\"\")"=w301) -> ("States Out"=w300:string)  [unwired: 14 in]
      }
      frame "Macro: Initialize" {
        # "Initialization Macro\n(This is called once, when the VI starts)"
        n127 = call <vilib>:"Add State(s) to Queue__JKI_lib_State_Machine.vi"("State(s) in Front (\"\")"="Data: Initialize\nInitialize Core Data\nUI: Initialize\nUI: Front Panel State >> Open\nData: UpdateStepSize\nUI: StartUp\nUI: Cursor Set >> Busy\nStage: Initialize\nUI: Update\nStage: Reset\nStage: Config\nUI: Cursor Set >> Idle\nStage: Home\nStage: GoToZero\nUI: Update", "State(s) in (\"\")"=w302) -> ("States Out"=w307:string)  [unwired: 13 in]
      }
      frame "Macro: Exit" {
        # "Exit Macro\n(This is called once, when the VI exits)"
        n128 = Unbundle By Name(w316) -> ("Core.Close Panel on Exit?"=w315:bool)
        n129 = Select(t="UI: Front Panel State >> Close", s=w315, f="") -> (s? t:f=w312:string)
        n130 = call <vilib>:"Add State(s) to Queue__JKI_lib_State_Machine.vi"("State(s) in Front (\"\")"="Stage: Close\nUI: Update" ("State(s) in Front (\"\")"), "State(s) in (\"\")"=w312, "State(s) at Back (\"\")"="Data: Cleanup\nExit") -> ("States Out"=w310:string)  [unwired: 12 in]
        n131 = call <vilib>:"Add State(s) to Queue__JKI_lib_State_Machine.vi"("State(s) in Front (\"\")"=w310, "State(s) in (\"\")"=w319) -> ("States Out"=w318:string)  [unwired: 13 in]
      }
      frame "---------- Core ----------" {
        # "Do not put any code in this frame.\n(it is a separator no-op)"
        n132 = call <vilib>:"Add State(s) to Queue__JKI_lib_State_Machine.vi"("State(s) in (\"\")"=w324) -> ("States Out"=w323:string)  [unwired: 14 in]
      }
      frame Default {
        w335 = 42 items=["No error", "Argument error", "Memory is full", "Out of zone", "End of file", "File already open", "Generic file I/O error", "File not found", "File permission error", "Disk is full", "Duplicate path", "Too many files open", "System feature not enabled", "Resource file not found", "Cannot add resource", "Resource not found", "Image not found", "Image memory error", "Pen does not exist", "Config type invalid", "Config token not found", "Config parse error", "Config memory error", "Bad external code format", "Bad external code offset", "External code not present", "Null window", "Destroy window error", "Null menu", "Print aborted", "Bad print record", "Print driver error", "Windows error during printing", "Memory error during printing", "Print dialog error", "Generic print error", "Invalid device refnum", "Device not found", "Device parameter error", "Device unit error", "Cannot open device", "Device call aborted", "Generic error", "Cancelled by user", "Object ID too low", "Object ID too high", "Object not in heap", "Unknown heap", "Unknown object (invalid DefProc)", "Unknown object (DefProc not in table)", "Message out of range", "Invalid (null) method", "Unknown message", "Manager call not supported", "Bad address", "Network operation in progress", "Network operation timed out", "Connection is busy", "Network attribute not supported", "Network error", "Address in use", "System out of memory", "Connection aborted", "Connection refused", "Not connected", "Already connected", "Connection closed", "Initialization error (interapplication manager)", "Bad occurrence", "Wait on unbound occurrence handler", "Occurrence queue overflow", "Datalog type conflict", "Unused", "Unrecognized type (interapplication manager)", "Memory corrupt", "Failed to make temporary DLL", "Old CIN version", "Drag socket not found", "Failed to load drop-object", "Failed to register OLE object", "Failed to release OLE object", "Format specifier type mismatch", "Unknown format specifier", "Too few format specifiers", "Too many format specifiers", "Scan failed", "Newer CIN version", "Error converting to variant", "Runtime menu error", "Password tampered", "Variant attribute not found", "Incompatible variant data type", "Event data is not available", "Event Store is not present", "Occurrence is not found", "Event Queue is not created", "Event info is not available", "Refnum passed is NULL", "Error retrieving Class GUID", "Error retrieving CoClass GUID", "Error retrieving TypeLib GUID.", "Bad built application magic bytes.", "Specific driver is different from the specific driver associated with the Logical Name.", "There is no session opened to the class driver.", "Max Error", "MAX - Error with config objects", "MAX - Error loading configuration", "MAX - Group not supported"]
        # "Current State"
        # "Do not delete, rename, or modify this frame.\n(this is used to capture unhandled states and typos)"
        # "Handle mistyped state name (developer tool)"
        n133 = Format Into String(format string="Software Exception: Unhandled State \"%s\"." ("message"), error in=w331, w326) -> (resulting string=w334:string, error out=w333:errorcluster)  [unwired: 1 in]
        n134 = call <vilib>:"Error Cluster From Error Code.vi"("show call chain? (False)"=TRUE, "error in (no error)"=w333, "error message (\"\")"=w334, "error code (0)"=w335) -> ("error out"=w332:errorcluster)  [unwired: 5 in]
        n135 = call <vilib>:"Add State(s) to Queue__JKI_lib_State_Machine.vi"("State(s) in (\"\")"=w330) -> ("States Out"=w329:string)  [unwired: 14 in]
      }
      frame "Initialize Core Data" {
        # "Do not delete, rename, or modify this frame.\n(this is used to determine panel behavior on exit)"
        # "originally closed?"
        # "exe?"
        # "If panel starts closed or is an EXE, then close it when we exit"
        n136 = property class="VI"() -> ("FP.State"=w340:T4)  [unwired: 2 in, 2 out]
        n137 = property class="App"() -> ("App.Kind"=w346:T5)  [unwired: 2 in, 2 out]
        n138 = control-ref of="Current VI Reference"() -> (w341:refnum<vi>)
        n139 = Equal?(x=w340, y=T4."Closed" ("Front Panel Window:State")) -> (x = y?=w338:bool)
        n140 = Equal?(x=w346, y=T5."Run Time System" ("Application:Kind")) -> (x = y?=w344:bool)
        n141 = Or(x=w338, y=w344) -> (x .or. y?=w342:bool)
        n142 = Bundle By Name(cluster=w343, "Core.Current VI Reference"=w341, "Core.Close Panel on Exit?"=w342) -> (w348:T6)
        n143 = call <vilib>:"Add State(s) to Queue__JKI_lib_State_Machine.vi"("State(s) in (\"\")"=w350) -> ("States Out"=w349:string)  [unwired: 14 in]
      }
      frame "Error Handler" {
        # "Unhandled Error -- Display it"
        # "Handle any errors here.\nYou can also output any states to clean-up after errors occur"
        # "Clear error"
        n144 = call <vilib>:"General Error Handler.vi"("error in (no error)"=w353) -> ()  [unwired: 10 in, 5 out]
        n145 = call <vilib>:"Add State(s) to Queue__JKI_lib_State_Machine.vi"("State(s) in Front (\"\")"="/* Post Error States\nMacro: Exit", "State(s) in (\"\")"=w357) -> ("States Out"=w356:string)  [unwired: 13 in]
      }
      frame "Exit" {
        # "Do not put any code in this frame.\n(No errors that occur here will be handled.)"
        n146 = Generate User Event(user event=w361, event data cluster=TRUE ("event data"), error in=w359) -> (error out=w360:errorcluster)  [unwired: 1 in, 1 out]
        n147 = call <vilib>:"Add State(s) to Queue__JKI_lib_State_Machine.vi"("State(s) in (\"\")"=w366) -> ("States Out"=w365:string)  [unwired: 14 in]
      }
      frame "---------- Data ----------" {
        # "Do not put any code in this frame.\n(It is a separator no-op. You can make a copy of this frame to create a new Data frame)"
        n148 = call <vilib>:"Add State(s) to Queue__JKI_lib_State_Machine.vi"("State(s) in (\"\")"=w371) -> ("States Out"=w370:string)  [unwired: 14 in]
      }
      frame "Data: Initialize" {
        w372 = FALSE  # StageStatus
        w373 = path ""  # SaveFilePath
        w375 = cluster{"X":sgl, "Y":sgl, "Z":sgl} {"X"=0.0, "Y"=0.0, "Z"=0.0}  # HomeMposOrigin
        w376 = FALSE  # StageHomed?
        w377 = 0.0  # YPixelSize(mm)
        w378 = 0  # Tic
        w379 = cluster{"X":sgl, "Y":sgl, "Z":sgl} {"X"=0.0, "Y"=0.0, "Z"=0.0}  # ScanOrigin
        w380 = 5.0  # StepSize
        w381 = refnum<visa-resource-name> "COM3"  # StageCOM
        w382 = T8 {"Current VI Reference"=refnum, "Close Panel on Exit?"=FALSE}  # Core
        # "Initialize the shift-register data, here.\n(data names are defined by what you wire into the bundle function)"
        n149 = Bundle("Core"=w382, "StageStatus"=w372, "StageCOM"=w381, "StepSize"=w380, "ScanOrigin"=w379, "HomeMposOrigin"=w375, "Tic"=w378, "YPixelSize(mm)"=w377, "StageHomed?"=w376, "SaveFilePath"=w373) -> (w384:T6)  [unwired: 1 in]
        n150 = call <vilib>:"Add State(s) to Queue__JKI_lib_State_Machine.vi"("State(s) in (\"\")"=w386) -> ("States Out"=w385:string)  [unwired: 14 in]
      }
      frame "Data: UpdateStepSize" {
        # "Template Separator\n(You can make a copy of, or modify, this frame)"
        n151 = Bundle By Name(cluster=w389, "StepSize"="Jog Step Size(mm)") -> (w390:T6)
        n152 = call <vilib>:"Add State(s) to Queue__JKI_lib_State_Machine.vi"("State(s) in (\"\")"=w393) -> ("States Out"=w392:string)  [unwired: 14 in]
      }
      frame "Data: Cleanup" {
        # "Cleanup any data and references, here.\n(this is called automatically, by the Macro: Exit)"
        n153 = Unbundle By Name(w395) -> ("Core.Current VI Reference"=w398:refnum<vi>)
        n154 = Close Reference(reference=w398, error in (no error)=w397) -> (error out=w396:errorcluster)
        n155 = call <vilib>:"Add State(s) to Queue__JKI_lib_State_Machine.vi"("State(s) in (\"\")"=w400) -> ("States Out"=w399:string)  [unwired: 14 in]
      }
      frame "---------- UI ----------" {
        # "Do not put any code in this frame.\n(It is a separator no-op. You can make a copy of this frame to create a new UI frame)"
        n156 = call <vilib>:"Add State(s) to Queue__JKI_lib_State_Machine.vi"("State(s) in (\"\")"=w405) -> ("States Out"=w404:string)  [unwired: 14 in]
      }
      frame "UI: StartUp" {
        w406 = T9."Disabled and Grayed Out" ("Disabled")
        # "Do not put any code in this frame.\n(It is a separator no-op. You can make a copy of this frame to create a new UI frame)"
        n157 = property on="Stage COM port" class="VISAName"("DisabledEnum"=w406) -> ()  [unwired: 2 in, 2 out]
        n158 = property on="RasterScan" class="Bool"("DisabledEnum"=w406) -> ()  [unwired: 2 in, 2 out]
        n159 = local write "Tab Control"(enum32{"Stage Control", "Stage Setting"}."Stage Setting" ("Tab Control")) -> ()
        n160 = property on="X-Axis configuration" class="Clust (strict)"("DisabledEnum"=w406) -> ()  [unwired: 2 in, 2 out]
        n161 = property on="Y-Axis configuration" class="Clust (strict)"("DisabledEnum"=w406) -> ()  [unwired: 2 in, 2 out]
        n162 = property on="Z-Axis configuration" class="Clust (strict)"("DisabledEnum"=w406) -> ()  [unwired: 2 in, 2 out]
        n163 = property on="Set Origin" class="Bool"("DisabledEnum"=w406) -> ()  [unwired: 2 in, 2 out]
        n164 = property on="Poll grbl position?" class="Bool (strict)"("DisabledEnum"=w406) -> ()  [unwired: 2 in, 2 out]
        n165 = property on="X++" class="Bool"("DisabledEnum"=w406) -> ()  [unwired: 2 in, 2 out]
        n166 = property on="X--" class="Bool"("DisabledEnum"=w406) -> ()  [unwired: 2 in, 2 out]
        n167 = property on="Y++" class="Bool"("DisabledEnum"=w406) -> ()  [unwired: 2 in, 2 out]
        n168 = property on="Y--" class="Bool"("DisabledEnum"=w406) -> ()  [unwired: 2 in, 2 out]
        n169 = property on="Z++" class="Bool"("DisabledEnum"=w406) -> ()  [unwired: 2 in, 2 out]
        n170 = property on="Z--" class="Bool"("DisabledEnum"=w406) -> ()  [unwired: 2 in, 2 out]
        n171 = property on="Hault" class="Bool"("DisabledEnum"=w406) -> ()  [unwired: 2 in, 2 out]
        n172 = property on="GoToZero" class="Bool"("DisabledEnum"=w406) -> ()  [unwired: 2 in, 2 out]
        n173 = property on="Home" class="Bool"("DisabledEnum"=w406) -> ()  [unwired: 2 in, 2 out]
        n174 = call <vilib>:"Add State(s) to Queue__JKI_lib_State_Machine.vi"("State(s) in (\"\")"=w412) -> ("States Out"=w411:string)  [unwired: 14 in]
      }
      frame "UI: Exit" {
        w413 = T9."Enabled" ("Disabled")
        # "Do not put any code in this frame.\n(It is a separator no-op. You can make a copy of this frame to create a new UI frame)"
        n175 = property on="Stage COM port" class="VISAName"("DisabledEnum"=w413) -> ()  [unwired: 2 in, 2 out]
        n176 = property on="X-Axis configuration" class="Clust (strict)"("DisabledEnum"=w413) -> ()  [unwired: 2 in, 2 out]
        n177 = property on="Y-Axis configuration" class="Clust (strict)"("DisabledEnum"=w413) -> ()  [unwired: 2 in, 2 out]
        n178 = property on="Z-Axis configuration" class="Clust (strict)"("DisabledEnum"=w413) -> ()  [unwired: 2 in, 2 out]
        n179 = call <vilib>:"Add State(s) to Queue__JKI_lib_State_Machine.vi"("State(s) in (\"\")"=w418) -> ("States Out"=w417:string)  [unwired: 14 in]
      }
      frame "UI: SysReady" {
        # "System finished start up and ready for use\n(It is a separator no-op. You can make a copy of this frame to create a new UI frame)"
        n180 = call <vilib>:"Add State(s) to Queue__JKI_lib_State_Machine.vi"("State(s) in (\"\")"=w423) -> ("States Out"=w422:string)  [unwired: 14 in]
      }
      frame "UI: Update" {
        # "Do not put any code in this frame.\n(It is a separator no-op. You can make a copy of this frame to create a new UI frame)"
        n181 = Unbundle By Name(w427) -> ("StageStatus"=w424:bool, "StageHomed?"=w425:bool)
        n182 = case shown="True" w425 {
          frame False {
          }
          frame True {
            w431 = T9."Enabled" ("Disabled")
            n183 = property on="GoToZero" class="Bool"("DisabledEnum"=w431) -> ()  [unwired: 2 in, 2 out]
            n184 = property on="RasterScan" class="Bool"("DisabledEnum"=w431) -> ()  [unwired: 2 in, 2 out]
          }
        }
        n185 = case shown="True" w424 {
          frame False {
          }
          frame True {
            w432 = T9."Enabled" ("Disabled")
            n186 = property on="Set Origin" class="Bool"("DisabledEnum"=w432) -> ()  [unwired: 2 in, 2 out]
            n187 = property on="Poll grbl position?" class="Bool (strict)"("DisabledEnum"=w432) -> ()  [unwired: 2 in, 2 out]
            n188 = property on="X++" class="Bool"("DisabledEnum"=w432) -> ()  [unwired: 2 in, 2 out]
            n189 = property on="X--" class="Bool"("DisabledEnum"=w432) -> ()  [unwired: 2 in, 2 out]
            n190 = property on="Y++" class="Bool"("DisabledEnum"=w432) -> ()  [unwired: 2 in, 2 out]
            n191 = property on="Y--" class="Bool"("DisabledEnum"=w432) -> ()  [unwired: 2 in, 2 out]
            n192 = property on="Z++" class="Bool"("DisabledEnum"=w432) -> ()  [unwired: 2 in, 2 out]
            n193 = property on="Z--" class="Bool"("DisabledEnum"=w432) -> ()  [unwired: 2 in, 2 out]
            n194 = property on="Hault" class="Bool"("DisabledEnum"=w432) -> ()  [unwired: 2 in, 2 out]
            n195 = property on="Home" class="Bool"("DisabledEnum"=w432) -> ()  [unwired: 2 in, 2 out]
          }
        }
        n196 = call <vilib>:"Add State(s) to Queue__JKI_lib_State_Machine.vi"("State(s) in (\"\")"=w430) -> ("States Out"=w429:string)  [unwired: 14 in]
      }
      frame "UI: Initialize" {
        # "Initialize the User Interface, here.\n(this is called automatically, by the Macro: Init)"
        n197 = call <vilib>:"Add State(s) to Queue__JKI_lib_State_Machine.vi"("State(s) in (\"\")"=w437) -> ("States Out"=w436:string)  [unwired: 14 in]
      }
      frame "UI: Cursor Set" {
        # "Argument"
        # "Set and Unset Cursor Busy.\n(Usage: \"UI: Cursor Set >> Busy|Idle\")"
        n198 = case shown="\"Idle\", Default" w439 {
          tunnel: w441 -> [w446 w448]
          tunnel: [w445 w447] -> w440
          frame "Idle", Default {
            n199 = call <vilib>:"Unset Busy.vi"("error in (no error)"=w446) -> ("error out"=w445:errorcluster)  [unwired: 10 in]
          }
          frame "Busy" {
            n200 = call <vilib>:"Set Busy.vi"("error in (no error)"=w448) -> ("error out"=w447:errorcluster)  [unwired: 9 in, 1 out]
          }
        }
        n201 = call <vilib>:"Add State(s) to Queue__JKI_lib_State_Machine.vi"("State(s) in (\"\")"=w444) -> ("States Out"=w443:string)  [unwired: 14 in]
      }
      frame "UI: Front Panel State" {
        # "Argument"
        # "Set Front Panel Open or Closed\n(Usage: \"UI: Front Panel State >> Open|Close\")"
        n202 = Unbundle By Name(w452) -> ("Core.Current VI Reference"=w451:refnum<vi>)
        n203 = case shown="\"Open\", \"Standard\", Default" w450 {
          tunnel: w454 -> [w462 w477 w488 w501 w514]
          tunnel: [w464 w478 w490 w503 w516] -> w453
          tunnel: w451 -> [w463 w475 w489 w502 w515]
          frame "Open", "Standard", Default {
            w457 = T4."Standard" ("State")
            n204 = property class="VI"(reference=w463, error in=w462) -> (reference out=w460:refnum<vi>, error out=w461:errorcluster, "FP.State"=w459:T4)
            n205 = Not Equal?(x=w459, y=w457) -> (x != y?=w458:bool)
            n206 = case shown="True" w458 {
              tunnel: [w468 w470] -> w464
              tunnel: w461 -> [w467 w470]
              tunnel: w460 -> [w466 _]
              tunnel: w457 -> [w465 _]
              frame True {
                n207 = invoke class="VI" method="FP.Open"(reference=w466, error in=w467, "Activate"=TRUE, "State"=w465) -> (error out=w468:errorcluster)  [unwired: 1 in, 4 out]
              }
              frame False {
              }
            }
          }
          frame "Close", "Closed" {
            n208 = property class="VI"(reference=w475, error in=w477) -> (reference out=w474:refnum<vi>, error out=w476:errorcluster, "FP.State"=w472:T4)
            n209 = Not Equal?(x=w472, y=T4."Closed" ("Front Panel Window:State")) -> (x != y?=w471:bool)
            n210 = case shown="True" w471 {
              tunnel: [w479 w482] -> w478
              tunnel: w476 -> [w479 w481]
              tunnel: w474 -> [_ w480]
              frame False {
              }
              frame True {
                n211 = invoke class="VI" method="FP.Close"(reference=w480, error in=w481) -> (error out=w482:errorcluster)  [unwired: 1 in, 2 out]
              }
            }
          }
          frame "Hidden", "Hide" {
            w483 = T4."Hidden" ("State")
            n212 = property class="VI"(reference=w489, error in=w488) -> (reference out=w486:refnum<vi>, error out=w487:errorcluster, "FP.State"=w485:T4)
            n213 = Not Equal?(x=w485, y=w483) -> (x != y?=w484:bool)
            n214 = case shown="True" w484 {
              tunnel: [w494 w495] -> w490
              tunnel: w487 -> [w493 w495]
              tunnel: w486 -> [w492 _]
              tunnel: w483 -> [w491 _]
              frame True {
                n215 = invoke class="VI" method="FP.Open"(reference=w492, error in=w493, "State"=w491) -> (error out=w494:errorcluster)  [unwired: 2 in, 4 out]
              }
              frame False {
              }
            }
          }
          frame "Minimize", "Minimized" {
            w496 = T4."Minimized" ("State")
            n216 = property class="VI"(reference=w502, error in=w501) -> (reference out=w499:refnum<vi>, error out=w500:errorcluster, "FP.State"=w498:T4)
            n217 = Not Equal?(x=w498, y=w496) -> (x != y?=w497:bool)
            n218 = case shown="True" w497 {
              tunnel: [w507 w508] -> w503
              tunnel: w500 -> [w506 w508]
              tunnel: w499 -> [w505 _]
              tunnel: w496 -> [w504 _]
              frame True {
                n219 = invoke class="VI" method="FP.Open"(reference=w505, error in=w506, "State"=w504) -> (error out=w507:errorcluster)  [unwired: 2 in, 4 out]
              }
              frame False {
              }
            }
          }
          frame "Maximize", "Maximized" {
            w509 = T4."Maximized" ("State")
            n220 = property class="VI"(reference=w515, error in=w514) -> (reference out=w512:refnum<vi>, error out=w513:errorcluster, "FP.State"=w511:T4)
            n221 = Not Equal?(x=w511, y=w509) -> (x != y?=w510:bool)
            n222 = case shown="True" w510 {
              tunnel: [w520 w521] -> w516
              tunnel: w513 -> [w519 w521]
              tunnel: w512 -> [w518 _]
              tunnel: w509 -> [w517 _]
              frame True {
                n223 = invoke class="VI" method="FP.Open"(reference=w518, error in=w519, "State"=w517) -> (error out=w520:errorcluster)  [unwired: 2 in, 4 out]
              }
              frame False {
              }
            }
          }
        }
        n224 = call <vilib>:"Add State(s) to Queue__JKI_lib_State_Machine.vi"("State(s) in (\"\")"=w456) -> ("States Out"=w455:string)  [unwired: 14 in]
      }
      frame "---------- Stage ----------" {
        # "Template Separator\n(You can make a copy of, or modify, this frame)"
        n225 = call <vilib>:"Add State(s) to Queue__JKI_lib_State_Machine.vi"("State(s) in (\"\")"=w526) -> ("States Out"=w525:string)  [unwired: 14 in]
      }
      frame "Stage: Initialize" {
        # "Initialize stage controler\n(Open connection and check)"
        n226 = call "Initialize Serial Port.vi"("VISA resource name"="Stage COM port", "baud rate (115200)"=u32 115200, "error in (no error)"=w536) -> ("error out"=w533:errorcluster)  [unwired: 12 in]
        n227 = call "Get Version.vi"("error in (no error)"=w533) -> ("Version information"=→"Version information":string, "error out"=w527:errorcluster)  [unwired: 12 in, 1 out]
        n228 = case shown="No Error" w527 {
          selector: w527 -> [w539 _]
          tunnel: [w539 w540] -> w532
          frame No Error {
          }
          frame Error {
            # "If grbl respond is wrong"
            n229 = xnode "Error Ring"() -> ("error out"=w540:errorcluster)
          }
        }
        n230 = case shown="No Error" w527 {
          tunnel: [w548 w550] -> w535
          tunnel: w528 -> [w547 w550]
          tunnel: "Stage COM port" -> [w546 _]
          frame No Error {
            n231 = Bundle By Name(cluster=w547, "StageStatus"=TRUE ("Sys Status.Stage"), "StageCOM"=w546) -> (w548:T6)
          }
          frame Error {
          }
        }
        n232 = call <vilib>:"Add State(s) to Queue__JKI_lib_State_Machine.vi"("State(s) in (\"\")"=w538) -> ("States Out"=w537:string)  [unwired: 14 in]
      }
      frame "Stage: Reset" {
        # "Reset grbl\n(Ctrl+x)"
        n233 = call "Reset.vi"("error in (no error)"=w552) -> ("error out"=w553:errorcluster)  [unwired: 14 in]
        n234 = call <vilib>:"Add State(s) to Queue__JKI_lib_State_Machine.vi"("State(s) in (\"\")"=w556) -> ("States Out"=w555:string)  [unwired: 14 in]
      }
      frame "Stage: Config" {
        w569 = T10 {"Invert enable pin"=FALSE, "Invert limit pin"=FALSE, "Invert probe pin"=FALSE}  # Pins direction
        w581 = T11 {"Reverse X"=TRUE, "Reverse Y"=TRUE, "Reverse Z"=FALSE}  # Homing direction invert
        w571 = T11 {"Reverse X"=FALSE, "Reverse Y"=FALSE, "Reverse Z"=FALSE}  # Step pulse invert
        w570 = T11 {"Reverse X"=TRUE, "Reverse Y"=TRUE, "Reverse Z"=FALSE}  # Axis direction
        # "set G code parser and default speed 2000"
        # "Initialize stage controler and set default configuration\n()"
        n235 = call "Config IO.vi"("Pulse time us"=u32 3, "Soft limit enable"=FALSE, "Hard limit enable"=FALSE, "Step idle delay ms (255 keep)"=u8 25, "Step pulse invert"=w571, "Axis direction"=w570, "error in (no error)"=w567, "Pins direction"=w569) -> ("error out"=w585:errorcluster)  [unwired: 7 in]
        n236 = call "Config Axis.vi"("X-Axis configuration"="X-Axis configuration", "Y-Axis configuration"="Y-Axis configuration", "Z-Axis configuration"="Z-Axis configuration", "error in (no error)"=w585) -> ("error out"=w584:errorcluster)  [unwired: 11 in]
        n237 = call "Config Home.vi"("Homing direction invert"=w581, "Homing cycle enable"=TRUE, "Homing locate feed rate\tmm/min"=u32 100 ("Homing locate feed rate\tmm/min"), "Homing search seek rate\tmm/min"=u32 3000 ("Homing search seek rate\tmm/min"), "Homing switch debounce delay\tms"=u32 25 ("Homing switch debounce delay\tms"), "error in (no error)"=w584, "Homing switch pull-off distance\tmm"=u32 2 ("Homing switch pull-off distance\tmm")) -> ("error out"=w583:errorcluster)  [unwired: 8 in]
        n238 = call "Release Lock from Alarm.vi"("error in (no error)"=w583) -> ("error out"=w582:errorcluster)  [unwired: 14 in]
        n239 = call "Get Configuration.vi"("error in (no error)"=w582) -> ("Config"=→"Current Config":string, "error out"=w563:errorcluster)  [unwired: 13 in]
        n240 = Concatenate Strings("G1F2000" ("Data to write"), "\r") -> (w559:string)
        n241 = call "Send-Receive Serial Port.vi"("Data to write"=w559, "error in (no error)"=w563) -> ("error out"=w562:errorcluster)  [unwired: 12 in, 1 out]
        n242 = call <vilib>:"Add State(s) to Queue__JKI_lib_State_Machine.vi"("State(s) in (\"\")"=w587) -> ("States Out"=w586:string)  [unwired: 14 in]
      }
      frame "Stage: Home" {
        # "Home Stage\n(You can make a copy of, or modify, this frame)"
        n243 = Two Button Dialog(message="Stage will home, please retrack fiber probe and make sure no object is in its way!", 1:"Cancel" ("F button name (\"Cancel\")"), 2:"Confirm" ("T button name (\"OK\")")) -> (T button?=w588:bool)
        n244 = case shown="True" w588 {
          tunnel: [w602 w612] -> w596
          tunnel: [w601 w611] -> w595
          tunnel: w594 -> [w601 w610]
          tunnel: w592 -> [w602 w609]
          frame False {
            n245 = One Button Dialog(message="You must home stage before doing any scanning! Some function of the program is now disabled!", button name ("OK")="Confirm") -> ()  [unwired: 1 out]
          }
          frame True {
            # "Update origin"
            n246 = call <vilib>:"Set Busy.vi"("error in (no error)"=w609) -> ("error out"=w604:errorcluster)  [unwired: 9 in, 1 out]
            n247 = call "Go home.vi"("Maximum wait time (45sec)"=30, "error in (no error)"=w604) -> ("error out"=w608:errorcluster)  [unwired: 13 in]
            n248 = call <vilib>:"Unset Busy.vi"("error in (no error)"=w608) -> ("error out"=w603:errorcluster)  [unwired: 10 in]
            n249 = Unbundle By Name(w608) -> ("status"=w607:bool)
            n250 = call "Get Status.vi"("error in (no error)"=w603) -> ("Current position"=w605:cluster{"X":sgl, "Y":sgl, "Z":sgl}, "error out"=w612:errorcluster)  [unwired: 10 in, 3 out]
            "Stage Home MPos" <- w605
            n251 = Not(x=w607) -> (.not. x?=w606:bool)
            n252 = local write "Current Machine Pos"(w605) -> ()
            n253 = Bundle By Name(cluster=w610, "StageHomed?"=w606, "HomeMposOrigin"=w605) -> (w611:T6)
          }
        }
        n254 = call <vilib>:"Add State(s) to Queue__JKI_lib_State_Machine.vi"("State(s) in (\"\")"=w598) -> ("States Out"=w597:string)  [unwired: 14 in]
      }
      frame "Stage: GoToZero" {
        # "Go to scanning origin marked on the platform\n(Go to scanning start and set original position)"
        n255 = Unbundle By Name(w615) -> ("StageHomed?"=w614:bool)
        n256 = case shown="True" w614 {
          tunnel: w619 -> [w625 w632]
          tunnel: [w625 w631] -> w618
          tunnel: [w624 w630] -> w617
          tunnel: w615 -> [w624 w628]
          frame False {
            # "stage not homed, do nothing"
            n257 = One Button Dialog(message="Stage not homed! Could not go to scan origin marked on stage platform! Please home stage and go to scan origin manually using the stage control.", button name ("OK")="Confirm") -> ()  [unwired: 1 out]
          }
          frame True {
            # "If stage is homed, move to scan origin"
            n258 = One Button Dialog(message="System will now go to scan starting point marked on the stage. Please make sure the stage is clear of any object.", button name ("OK")="Confirm" ("T button name (\"OK\")")) -> (true=w626:bool)
            n259 = case shown="True" w626 {
              tunnel: w632 -> [w634 w640]
              tunnel: [w634 w639] -> w631
              tunnel: [w633 w637] -> w630
              tunnel: w628 -> [w633 w635]
              frame False {
                # "user not confirmed, do nothing"
              }
              frame True {
                # "User confirm moving to scan origin"
                n260 = call "Get Status.vi"("error in (no error)"=w640) -> ("Status"=w644:T3, "error out"=w641:errorcluster)  [unwired: 10 in, 3 out]
                n261 = Equal?(x=Status."Idle" ("Status"), y=w644) -> (x = y?=w642:bool)
                n262 = case shown="True" w642 {
                  tunnel: w641 -> [w646 w655]
                  tunnel: [w646 w647] -> w638
                  frame False {
                    n263 = One Button Dialog(message="Could not go to starting point. ") -> ()  [unwired: 1 in, 1 out]
                  }
                  frame True {
                    n264 = call <vilib>:"Set Busy.vi"("error in (no error)"=w655) -> ("error out"=w648:errorcluster)  [unwired: 9 in, 1 out]
                    n265 = call "Go to Position.vi"("X (mm)"=sgl -150.0, "Speed (2000 mm/min)"=sgl 3000.0 ("Speed (mm/min)"), "Overwright speed? (F)"=TRUE, "Y (mm)"=sgl -150.0, "Z (mm)"=sgl 0.0, "error in (no error)"=w648) -> ("error out"=w651:errorcluster)  [unwired: 9 in]
                    n266 = call <vilib>:"Unset Busy.vi"("error in (no error)"=w651) -> ("error out"=w647:errorcluster)  [unwired: 10 in]
                  }
                }
                n267 = call "Get Status.vi"("error in (no error)"=w638) -> ("Current position"=w636:cluster{"X":sgl, "Y":sgl, "Z":sgl}, "error out"=w639:errorcluster)  [unwired: 10 in, 3 out]
                n268 = Bundle By Name(cluster=w635, "ScanOrigin"=w636) -> (w637:T6)
                n269 = local write "Scan Origin MPos"(w636) -> ()
              }
            }
          }
        }
        n270 = call <vilib>:"Add State(s) to Queue__JKI_lib_State_Machine.vi"("State(s) in (\"\")"=w621) -> ("States Out"=w620:string)  [unwired: 14 in]
      }
      frame "Stage: SendCommand" {
        # "Template Separator\n(You can make a copy of, or modify, this frame)"
        n271 = call "Send-Receive Serial Port.vi"("Data to write"=w657, "error in (no error)"=w658) -> ("error out"=w659:errorcluster)  [unwired: 12 in, 1 out]
        n272 = call <vilib>:"Add State(s) to Queue__JKI_lib_State_Machine.vi"("State(s) in (\"\")"=w662) -> ("States Out"=w661:string)  [unwired: 14 in]
      }
      frame "Stage: Close" {
        # "Close Stage connection\n(You can make a copy of, or modify, this frame)"
        n273 = Unbundle By Name(w664) -> ("StageStatus"=w663:bool)
        n274 = case shown="True" w663 {
          tunnel: [w672 w677] -> w668
          tunnel: w667 -> [w672 w676]
          tunnel: w664 -> [w671 w675]
          tunnel: [w671 w673] -> w666
          frame False {
          }
          frame True {
            n275 = call "Close Serial Port.vi"("error in (no error)"=w676) -> ("error out"=w677:errorcluster)  [unwired: 14 in]
            n276 = Bundle By Name(cluster=w675, "StageStatus"=FALSE ("Sys Status.Stage COM")) -> (w673:T6)
          }
        }
        n277 = call <vilib>:"Add State(s) to Queue__JKI_lib_State_Machine.vi"("State(s) in (\"\")"=w670) -> ("States Out"=w669:string)  [unwired: 14 in]
      }
      frame "---------- Utility ----------" {
        # "Template Separator\n(You can make a copy of, or modify, this frame)"
        n278 = call <vilib>:"Add State(s) to Queue__JKI_lib_State_Machine.vi"("State(s) in (\"\")"=w682) -> ("States Out"=w681:string)  [unwired: 14 in]
      }
      frame "Utility: Dewelling" {
        # "Template Separator\n(e.x. Dewelling >> 1000)"
        n279 = Decimal String To Number(string=w685) -> (number=w684:i32)  [unwired: 2 in, 1 out]
        n280 = Wait (ms)(milliseconds to wait=w684) -> ()  [unwired: 1 out]
        n281 = call <vilib>:"Add State(s) to Queue__JKI_lib_State_Machine.vi"("State(s) in (\"\")"=w689) -> ("States Out"=w688:string)  [unwired: 14 in]
      }
      frame "---------- New Category ----------" {
        # "Template Separator\n(You can make a copy of, or modify, this frame)"
        n282 = call <vilib>:"Add State(s) to Queue__JKI_lib_State_Machine.vi"("State(s) in (\"\")"=w694) -> ("States Out"=w693:string)  [unwired: 14 in]
      }
      frame "New Category: 1" {
        # "Your code here.\n(You can make a copy of, or modify, this frame)"
        n283 = call <vilib>:"Add State(s) to Queue__JKI_lib_State_Machine.vi"("State(s) in (\"\")"=w699) -> ("States Out"=w698:string)  [unwired: 14 in]
      }
      frame "New Category: 2" {
        # "Your code here.\n(You can make a copy of, or modify, this frame)"
        n284 = call <vilib>:"Add State(s) to Queue__JKI_lib_State_Machine.vi"("State(s) in (\"\")"=w704) -> ("States Out"=w703:string)  [unwired: 14 in]
      }
    }
  }
  n285 = while {
    tunnel: w14 -> [w709]
    tunnel: [w706] -> w13
    tunnel: w6 -> [w705]
    stop <- w707 stop-if-true
    # "Scan loop (both pre and follow)"
    n286 = event shown="[1] <3D profile scan pts>: User Event" {
      selector: w709 -> [_ _ _]
      dyn-events: [_ _ _] -> w706
      timeout: 10 -> [_ _ _]
      tunnel: [_ _ TRUE] -> w707
      tunnel: w705 -> [_ w712 _]
      event Timeout {
        n287 = event-data() -> ()  [unwired: 1 in, 3 out]
      }
      event User Event {
        w722 = "\r"
        n288 = event-data() -> ("3D profile scan pts"=w715:cluster{"x(mm)":dbl, "y(mm)":dbl, "z(mm)":dbl}[])  [unwired: 1 in, 4 out]
        n289 = flat-sequence {
          tunnel: w715 -> [w727]
          tunnel: [w727] -> w714
          frame #0 {
            n290 = Wait (ms)(milliseconds to wait=u32 100) -> ()  [unwired: 1 out]
          }
        }
        n291 = for {
          shift-right: [w732] -> w717
          shift-left: errorcluster {"status"=FALSE, "code"=0, "source"=""} ("error out") -> [w734]
          tunnel: w714 -> [w731] mode=indexing
          stop <- w732 stop-if-true
          n292 = Unbundle By Name(w731) -> ("x(mm)"=w730:dbl, "y(mm)"=w729:dbl, "z(mm)"=w728:dbl)
          n293 = Not A Number/Path/Refnum?(number/path/refnum=w728) -> (NaN/Path/Refnum?=w733:bool)
          n294 = case shown="False" w733 {
            tunnel: w734 -> [w739 w741]
            tunnel: [w738 w741] -> w732
            tunnel: w730 -> [w737 _]
            tunnel: w729 -> [w736 _]
            tunnel: w728 -> [w735 _]
            frame False {
              # "if z not NaN, send"
              n295 = call "Go to Position.vi"("X (mm)"=w737, "Y (mm)"=w736, "Z (mm)"=w735, "Wait for finish? (T)"=TRUE, "error in (no error)"=w739) -> ("error out"=w738:errorcluster)  [unwired: 10 in]
            }
            frame True {
              # "if z is NaN, do nothing"
            }
          }
        }
        n296 = while {
          shift-right: [w750] -> w713
          shift-left: w717 -> [w751]
          i -> [w745]
          stop <- w742 stop-if-true
          n297 = Greater?(x=w745, y=500) -> (0:w743:bool)
          n298 = call "Get Status.vi"("error in (no error)"=w751) -> ("Status"=w749:T3, "error out"=w750:errorcluster)  [unwired: 10 in, 3 out]
          n299 = Wait (ms)(milliseconds to wait=u32 100) -> ()  [unwired: 1 out]
          n300 = Equal?(x=Status."Idle" ("Status"), y=w749) -> (x = y?=w746:bool)
          n301 = Or(x=w746, y=w743) -> (x .or. y?=w742:bool)
        }
        n302 = Generate User Event(user event=w712, event data cluster=TRUE ("event data"), error in=w713) -> (error out=→"error out":errorcluster)  [unwired: 1 in, 1 out]
        n303 = Concatenate Strings("$120=500" ("string"), w722) -> (w721:string)
        n304 = Concatenate Strings("$121=200" ("string"), w722) -> (w720:string)
        n305 = Concatenate Strings("$122=500" ("string"), w722) -> (w719:string)
        n306 = Build Array(w721, w720, w719) -> (w718:string[])
        n307 = for {
          tunnel: w713 -> [w753]
          tunnel: w718 -> [w752] mode=indexing
          n308 = call "Send-Receive Serial Port.vi"("Data to write"=w752, "error in (no error)"=w753) -> ()  [unwired: 12 in, 2 out]
        }
      }
      event User Event {
        n309 = event-data() -> ()  [unwired: 1 in, 5 out]
      }
    }
  }
  n310 = local write "Poll grbl position?"(TRUE) -> ()
  n311 = Unregister For Events(event registration refnum=w7, error in=w1) -> (error out=w5:errorcluster)
  n312 = Unregister For Events(event registration refnum=w13, error in=w1) -> (error out=w12:errorcluster)
  n313 = Destroy User Event(user event=w6, error in=w5) -> (error out=w2:errorcluster)
  n314 = Destroy User Event(user event=w10, error in=w12) -> (error out=w11:errorcluster)
  n315 = Merge Errors(w2, w1, w11) -> (w20:errorcluster)
  n316 = call <vilib>:"Simple Error Handler.vi"("error in (no error)"=w20) -> ()  [unwired: 4 in, 5 out]
